vi "NI.History (Boolean).vi"(1 "value in":bool) -> (0 "Stop?":bool)   [LabVIEW 2020]
doc: "Displays the value of the 32-bit signed integer numeric control and allows conditional breakpoints."
uses:
  <vilib>/Utility/miscctls.llb/LVRowAndColumnUnsignedTypeDef.ctl
panel:
  out "History":i32(listbox)=-1
  in  "reset":bool
  # "* Changes take effect the next time the probe runs."
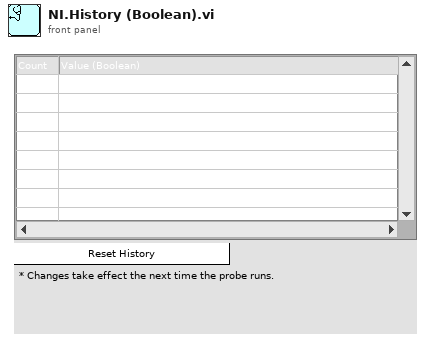
[diagram p1: front panel]
types:
  T1 = typedef "LVRowAndColumnUnsignedTypeDef.ctl" = cluster{"Row":u32, "Column":u32}
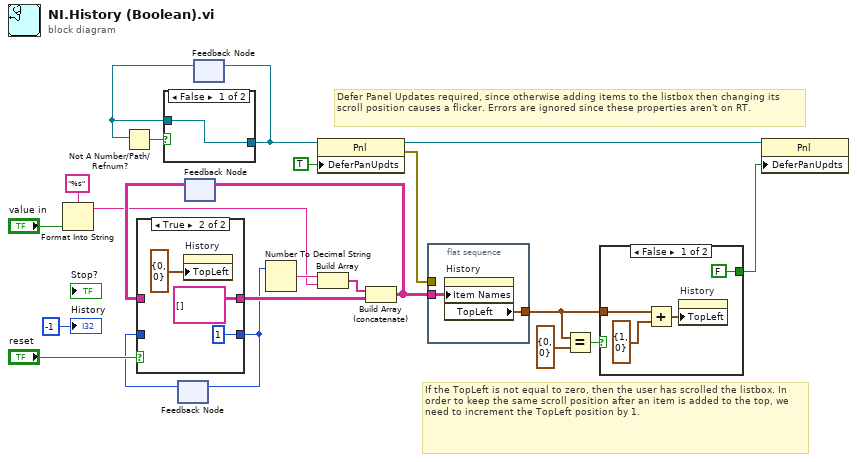
[diagram p0: block diagram]
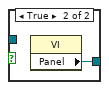
[diagram p2: hidden frame]
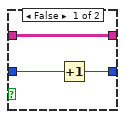
[diagram p4: hidden frame]
diagram:
  # "If the TopLeft is not equal to zero, then the user has scrolled the listbox. In order to keep the same scroll position after an item is added to the top, we need to increment the TopLeft position by 1."
  # "Defer Panel Updates required, since otherwise adding items to the listbox then changing its scroll position causes a flicker. Errors are ignored since these properties aren't on RT."
  n1 = Format Into String(format string="%s", "value in") -> (resulting string=w11:string)  [unwired: 2 in, 1 out]
  n2 = feedback #1() -> (w16:i32)  [unwired: 1 in]
  n3 = feedback #2() -> (w15:string[][])  [unwired: 1 in]
  n4 = case shown="True" "reset" {
    tunnel: w15 -> [w25 _]
    tunnel: w16 -> [w24 _]
    tunnel: [w25 string[][] []] -> w20
    tunnel: [w23 1] -> w17
    frame False {
      n5 = Increment(x=w24) -> (x+1=w23:i32)
    }
    frame True {
      n6 = property on="History" class="MCListbox (strict)"("TopLeft"=T1 {"Row"=0, "Column"=0} ("Top Left Visible Cell")) -> ()  [unwired: 2 in, 2 out]
    }
  }
  n7 = feedback-in #1(w17) -> ()
  n8 = feedback #3() -> (w7:refnum<vi>)  [unwired: 1 in]
  n9 = Not A Number/Path/Refnum?(number/path/refnum=w7) -> (NaN/Path/Refnum?=w8:bool)
  n10 = case shown="False" w8 {
    tunnel: [w29 w30] -> w9
    tunnel: w7 -> [w29 _]
    frame False {
    }
    frame True {
      n11 = property class="VI"() -> ("Panel"=w30:refnum<vi>)  [unwired: 2 in, 2 out]
    }
  }
  n12 = feedback-in #3(w9) -> ()
  n13 = Number To Decimal String(number=w17) -> (decimal integer string=w18:string)  [unwired: 1 in]
  n14 = property class="Pnl"(reference=w9, "DeferPanUpdts"=TRUE ("Defer Panel Updates")) -> (reference out=w6:refnum<vi>, error out=w2:errorcluster)  [unwired: 1 in]
  n15 = Build Array(w18, w11) -> (w19:string[])
  n16 = Build Array (concatenate)(w19, w20) -> (w14:string[][])
  n17 = feedback-in #2(w14) -> ()
  n18 = flat-sequence {
    tunnel: w14 -> [w32]
    tunnel: [w31] -> w3
    tunnel: w2 -> [_]
    frame #0 {
      n19 = property on="History" class="MCListbox (strict)"("Item Names"=w32) -> ("TopLeft"=w31:T1)  [unwired: 2 in, 2 out]
    }
  }
  n20 = Equal?(x=w3, y=T1 {"Row"=0, "Column"=0} ("Top Left Visible Cell")) -> (x = y?=w5:bool)
  n21 = case shown="False" w5 {
    tunnel: w3 -> [w36 _]
    tunnel: [FALSE ("Defer Panel Updates") _] -> w1
    frame False {
      n22 = Add(x=w36, y=T1 {"Row"=1, "Column"=0}) -> (x+y=w34:T1)
      n23 = property on="History" class="MCListbox (strict)"("TopLeft"=w34) -> ()  [unwired: 2 in, 2 out]
    }
    frame True {
    }
  }
  n24 = property class="Pnl"(reference=w6, "DeferPanUpdts"=w1) -> ()  [unwired: 1 in, 2 out]
  "History" <- -1 ("History of Values")
